vi "MotionProfileChange.vi"(7 "Motion Mode":enum16{"Move Mode", "Scan Mode"}(ring), 10 "Location":T5, 11 "Motion Settings In in":T1={"No Motion?"=FALSE, "Motion System"=enum."MM3000", "Motion Bd ID"=0, "Motion Profile"="", "# Axis"=0, "Reverse Z axis?"=FALSE, "SMAC Axis"=0, "scan pair"=enum."y-(x) scan", "RT fps"=0.0, "Steps per mm"=[], "Motor Parameters"={"velocity ct/s"=[], "accel ct/s^2"=[]}, "One Way Scan"=FALSE, "Reverse One Way Scan"=FALSE, "Global Position (mm)"=[], "Plane"=0, "Distance between\nscan lines (um)"=0.0, "Distance between\nscan planes (um)"=0.0, "number of scan planes"=0, "Total steps in line"=0, "Xtra plane\ndistance  (um)"=0, "Xtra planes "=0, "Add Axis"=FALSE, "overshoot cts"=0, "BKPT Shift"=0, "Scan Start Time (ms)"=0, "ESP VISA"="", "3rd Axis"=1, "GL Ref Out"=refnum, "Galil Address"=""} {"3rd Axis" items=["x", "y", "z", "w"]; "Xtra planes" min=1; "Xtra plane\ndistance  (um)" min=0; "Distance between\nscan planes (um)" format="%.2f"; "Distance between\nscan lines (um)" format="%.2f"; "SMAC Axis" items=["None"=0, "Axis 1"=1, "Axis 2"=2, "Axis 3"=3, "Axis 4"=4, "Axis 5"=5, "Axis 6"=6, "Axis 7"=7, "Axis 8"=8, "Vector Space 1"=17, "Vector Space 2"=18, "Vector Space 3"=19, "Vector Space 4"=20]; "Motion Bd ID" min=1 max=32 step=1}) -> (3 "Motion Settings In out":T1={"No Motion?"=FALSE, "Motion System"=enum."MM3000", "Motion Bd ID"=0, "Motion Profile"="", "# Axis"=0, "Reverse Z axis?"=FALSE, "SMAC Axis"=0, "scan pair"=enum."y-(x) scan", "RT fps"=0.0, "Steps per mm"=[], "Motor Parameters"={"velocity ct/s"=[], "accel ct/s^2"=[]}, "One Way Scan"=FALSE, "Reverse One Way Scan"=FALSE, "Global Position (mm)"=[], "Plane"=0, "Distance between\nscan lines (um)"=0.0, "Distance between\nscan planes (um)"=0.0, "number of scan planes"=0, "Total steps in line"=0, "Xtra plane\ndistance  (um)"=0, "Xtra planes "=0, "Add Axis"=FALSE, "overshoot cts"=0, "BKPT Shift"=0, "Scan Start Time (ms)"=0, "ESP VISA"="", "3rd Axis"=1, "GL Ref Out"=refnum, "Galil Address"=""} {"3rd Axis" items=["x", "y", "z", "w"]; "Xtra planes" min=1; "Xtra plane\ndistance  (um)" min=0; "Distance between\nscan planes (um)" format="%.2f"; "Distance between\nscan lines (um)" format="%.2f"; "SMAC Axis" items=["None"=0, "Axis 1"=1, "Axis 2"=2, "Axis 3"=3, "Axis 4"=4, "Axis 5"=5, "Axis 6"=6, "Axis 7"=7, "Axis 8"=8, "Vector Space 1"=17, "Vector Space 2"=18, "Vector Space 3"=19, "Vector Space 4"=20]; "Motion Bd ID" min=1 max=32 step=1})   [LabVIEW 2022 SP3]
uses:
  -ScanSystem/Controls/location.ctl
  NI_controller/-NI_MotionRoutines/MotionParameters.ctl
  NI_controller/-NI_MotionRoutines/MotionSys.ctl
  -MotionRoutines/ScanAxis.ctl
  -MotionRoutines/3rdAxis.ctl
  -MotionRoutines/MotionGlobals.vi
panel:
  # "1-D and 2-D B scan settings"
  # "1-D and 2-D B scan settings"
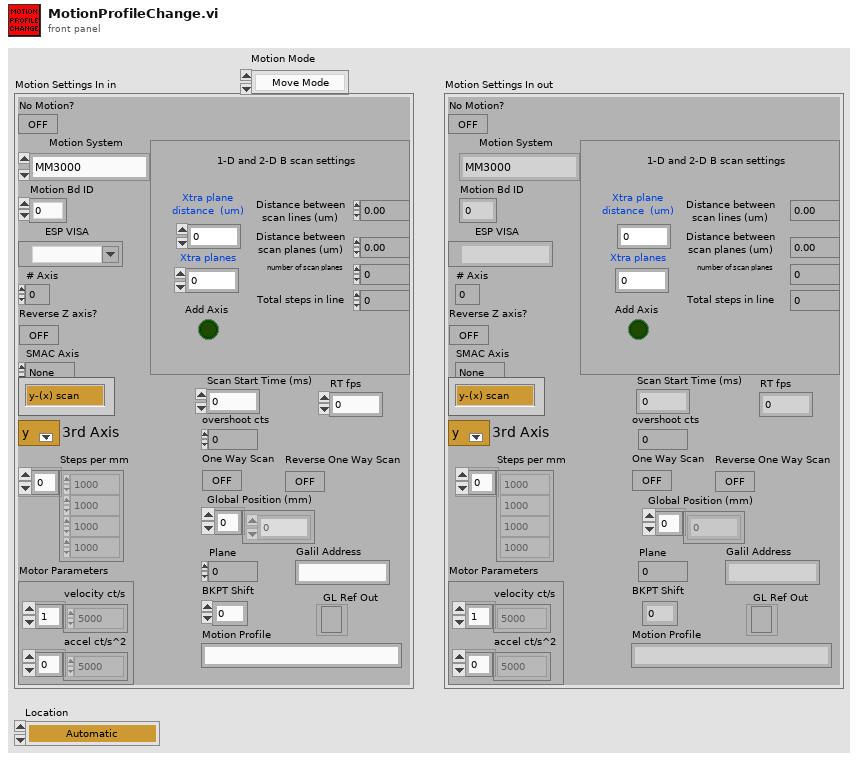
[diagram p1: front panel]
types:
  T1 = typedef "MotionParameters.ctl" = cluster{"No Motion?":bool, "Motion System":T2, "Motion Bd ID":u8, "Motion Profile":string, "# Axis":i8, "Reverse Z axis?":bool, "SMAC Axis":u16, "scan pair":T3, "RT fps":sgl, "Steps per mm":i32[], "Motor Parameters":cluster{"velocity ct/s":dbl[], "accel ct/s^2":dbl[]}, "One Way Scan":bool, "Reverse One Way Scan":bool, "Global Position (mm)":dbl[], "Plane":i32, "Distance between\nscan lines (um)":sgl, "Distance between\nscan planes (um)":sgl, "number of scan planes":i32, "Total steps in line":i32, "Xtra plane\ndistance  (um)":i32, "Xtra planes ":i32, "Add Axis":bool, "overshoot cts":i32, "BKPT Shift":i32, "Scan Start Time (ms)":u32, "ESP VISA":refnum<visa-resource-name>, "3rd Axis":T4, "GL Ref Out":refnum<k7>, "Galil Address":string}
  T2 = typedef "MotionSys.ctl" = enum16{"MM3000", "NI 735x", "Newport ESP", "No Motion Card", "Galil"}
  T3 = typedef "ScanAxis.ctl" = enum16{"y-(x) scan", "x-(y) scan", "z-(x) scan", "z-(y) scan", "y-(z) scan", "x-(z) scan", "w-(x) scan", "w-(y) scan", "w-(z) scan", "x-(w) scan", "y-(w) scan", "z-(w) scan"}
  T4 = typedef "3rdAxis.ctl" = u16
  T5 = typedef "location.ctl" = enum16{"Automatic", "WCM Main", "Hawaii", "Columbia MM3000", "Columbia  NI System", "NYU", "RRI 2", "UHI Allen", "CUMC RT", "Chiba", "Stony Brook", "WCM Microscopy", "WCM Aeoretch", "WCM Optics Lab", "WCM Main 2Axis", "WCM Rotation", "WCM SAM SMAC", "SERI GP"}
  T6 = typedef "EKG_Mode.ctl" = u16
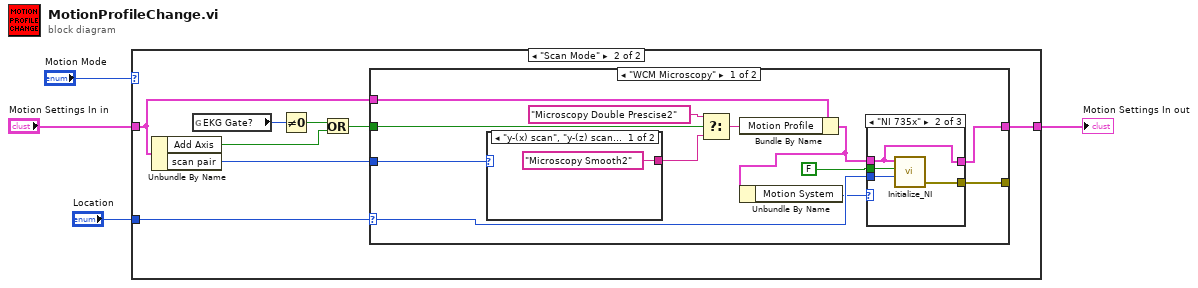
[diagram p0: block diagram]
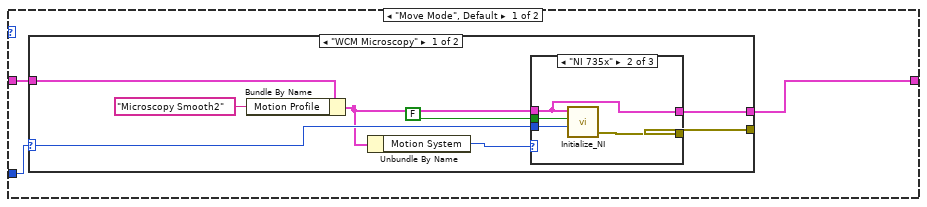
[diagram p2: hidden frame]
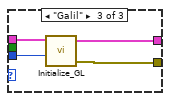
[diagram p4: hidden frame]
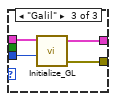
[diagram p7: hidden frame]
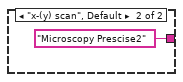
[diagram p8: hidden frame]
diagram:
  n1 = case shown="\"Scan Mode\"" "Motion Mode" {
    tunnel: "Location" -> [w7 w29]
    tunnel: [w5 w33] -> w3
    tunnel: "Motion Settings In in" -> [w6 w32]
    frame "Move Mode", Default {
      n2 = case shown="\"WCM Microscopy\"" w7 {
        selector: w7 -> [w14 _]
        tunnel: w6 -> [w13 w25]
        tunnel: [w12 _] -> _
        tunnel: [w8 w25] -> w5
        frame "WCM Microscopy" {
          n3 = Bundle By Name(cluster=w13, "Motion Profile"="Microscopy Smooth2") -> (w10:T1)
          n4 = Unbundle By Name(w10) -> ("Motion System"=w9:T2)
          n5 = case shown="\"NI 735x\"" w9 {
            tunnel: FALSE ("Bypass Init") -> [_ w20 _]
            tunnel: w14 -> [_ w19 w24]
            tunnel: w10 -> [w16 w17 w23]
            tunnel: [_ w18 w22] -> w12
            tunnel: [w16 w17 w21] -> w8
            frame "MM3000", Default {
            }
            frame "NI 735x" {
              n6 = call "Initialize_NI.vi"("Motion Settings"=w17, "Bypass Motion Init"=w20, "Location"=w19) -> ("error out"=w18:errorcluster)  [unwired: 2 in, 2 out]
            }
            frame "Galil" {
              n7 = call "Initialize_GL.vi"("Motion Settings"=w23, "Location"=w24) -> ("Motion Settings"=w21:T1, "error out"=w22:errorcluster)  [unwired: 3 in, 1 out]
            }
          }
        }
        frame "WCM Main", Default {
        }
      }
    }
    frame "Scan Mode" {
      n8 = Unbundle By Name(w32) -> ("Add Axis"=w31:bool, "scan pair"=w30:T3)
      n9 = global read "MotionGlobals.vi" "EKG Gate?"() -> (w26:T6)
      n10 = Not Equal To 0?(x=w26) -> (x != 0?=w27:bool)
      n11 = Or(x=w27, y=w31) -> (x .or. y?=w28:bool)
      n12 = case shown="\"WCM Microscopy\"" w29 {
        selector: w29 -> [w44 _]
        tunnel: w32 -> [w43 w57]
        tunnel: [w34 w57] -> w33
        tunnel: [w42 _] -> _
        tunnel: w30 -> [w41 _]
        tunnel: w28 -> [w38 _]
        frame "WCM Microscopy" {
          n13 = case shown="\"y-(x) scan\", \"y-(z) scan\", \"y-(w) scan\"" w41 {
            tunnel: ["Microscopy Smooth2" ("Motion Profile") "Microscopy Prescise2" ("Motion Profile")] -> w39
            frame "y-(x) scan", "y-(z) scan", "y-(w) scan" {
            }
            frame "x-(y) scan", Default {
            }
          }
          n14 = Select(t="Microscopy Double Prescise2" ("Motion Profile"), s=w38, f=w39) -> (s? t:f=w40:string)
          n15 = Bundle By Name(cluster=w43, "Motion Profile"=w40) -> (w36:T1)
          n16 = Unbundle By Name(w36) -> ("Motion System"=w35:T2)
          n17 = case shown="\"NI 735x\"" w35 {
            tunnel: FALSE ("Bypass Init") -> [_ w50 _]
            tunnel: w44 -> [_ w49 w54]
            tunnel: w36 -> [w46 w47 w53]
            tunnel: [_ w48 w52] -> w42
            tunnel: [w46 w47 w51] -> w34
            frame "MM3000", Default {
            }
            frame "NI 735x" {
              n18 = call "Initialize_NI.vi"("Motion Settings"=w47, "Bypass Motion Init"=w50, "Location"=w49) -> ("error out"=w48:errorcluster)  [unwired: 2 in, 2 out]
            }
            frame "Galil" {
              n19 = call "Initialize_GL.vi"("Motion Settings"=w53, "Location"=w54) -> ("Motion Settings"=w51:T1, "error out"=w52:errorcluster)  [unwired: 3 in, 1 out]
            }
          }
        }
        frame "WCM Main", Default {
        }
      }
    }
  }
  "Motion Settings In out" <- w3
